vi "Hypervisor_backup.vi"() -> ()   [LabVIEW 2014]
uses:
  Resource Type.ctl
  HypervisorState.ctl
  <vilib>/NI/Tools/String/Tools_String.lvlib
  <userlib>/_OpenG.lib/file/file.llb/Strip Path - Traditional__ogtk.vi
  Sensor Reading.ctl
  Resource.ctl
panel:
  out "Terminal":string
  in  "Module DataType 2":T1
  in  "Cancel Button":bool
  in  "Load Settings":bool
  in  "Module DataType":T1
  in  "Config File":path=path "C:/developer/New Model/config.txt"
  in  "Sensor Reading 3":T3
  in  "Sensor Reading 2":T3
  in  "Hypervisor State":T4=enum."Hypervisor.Sleeping"
  # "This is the hypervisor VI - it reads in a config file and loads the sub-VI's dictated in it asynchronously."
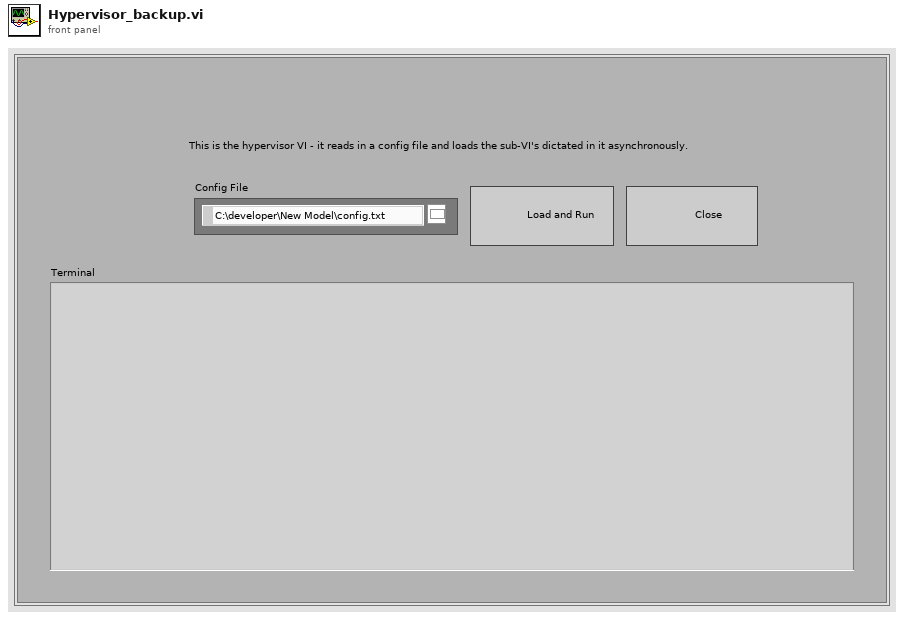
[diagram p1: front panel]
types:
  T1 = typedef "Resource.ctl" = cluster{"Module Name":string, "Message Queue":refnum<queue>, "Resource Type":T2, "Current State":enum16{"Invalid", "InMemory", "Running", "Paused", "Error", ""}, "Data Queue":refnum<queue>, "VI Reference":refnum<vi>}
  T2 = typedef "Resource Type.ctl" = enum16{"Consumer", "Producer", "Observer"}
  T3 = typedef "Sensor Reading.ctl" = cluster{"Sensor Name":string, "Timestamp":string, "Data Chunk":string}
  T4 = typedef "HypervisorState.ctl" = enum16{"Hypervisor.Error", "Hypervisor.Sleeping", "Hypervisor.Loaded", "Hypervisor.Booting", "Hypervisor.Testing", "Hypervisor.Calibrating", "Hypervisor.Running"}
  T5 = enum16{"Invalid", "InMemory", "Running", "Paused", "Error", ""}
  T6 = typedef "Config Data.ctl" = cluster{"Tower ID":string, "Access Password":string}
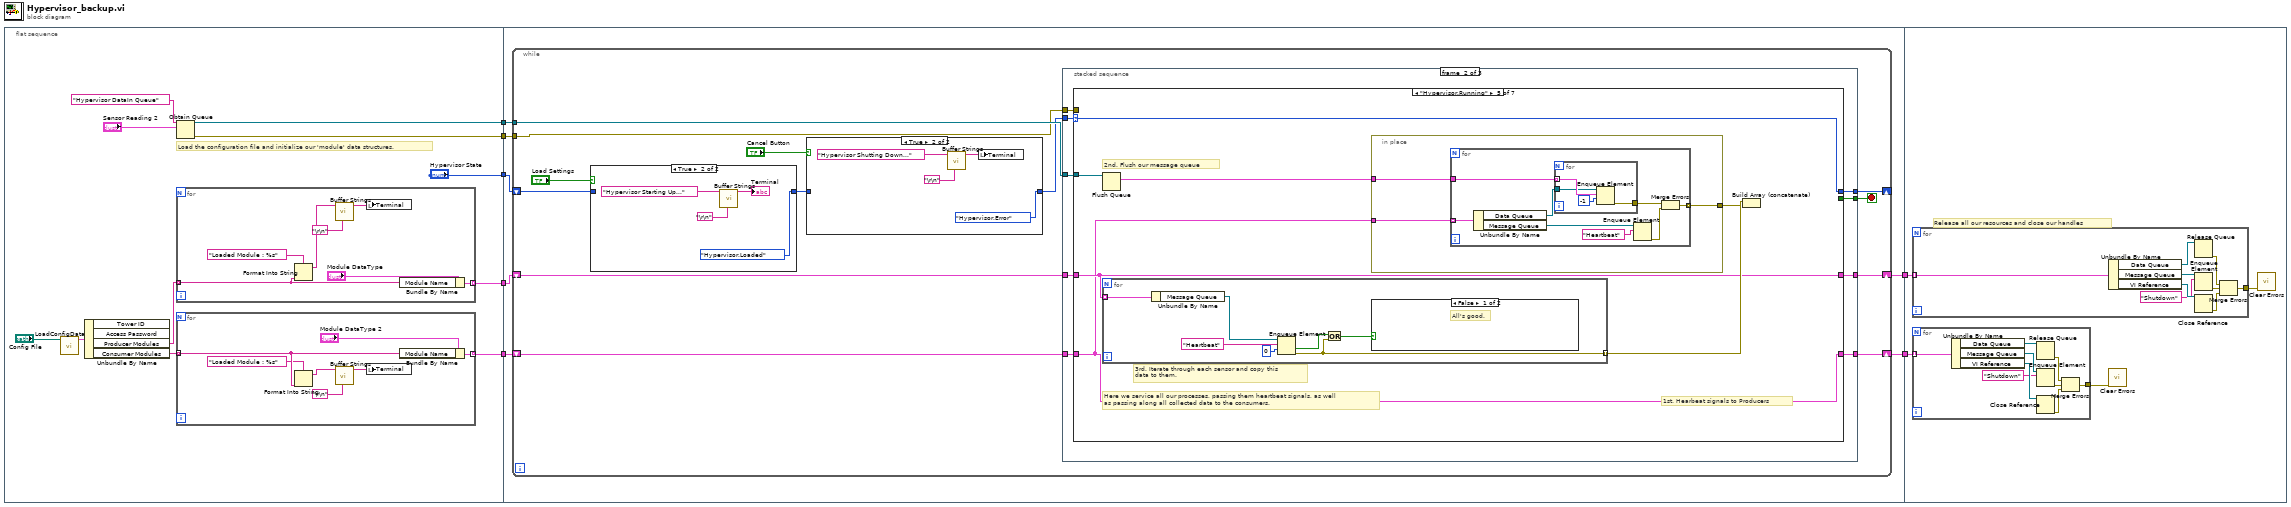
[diagram p0: block diagram]
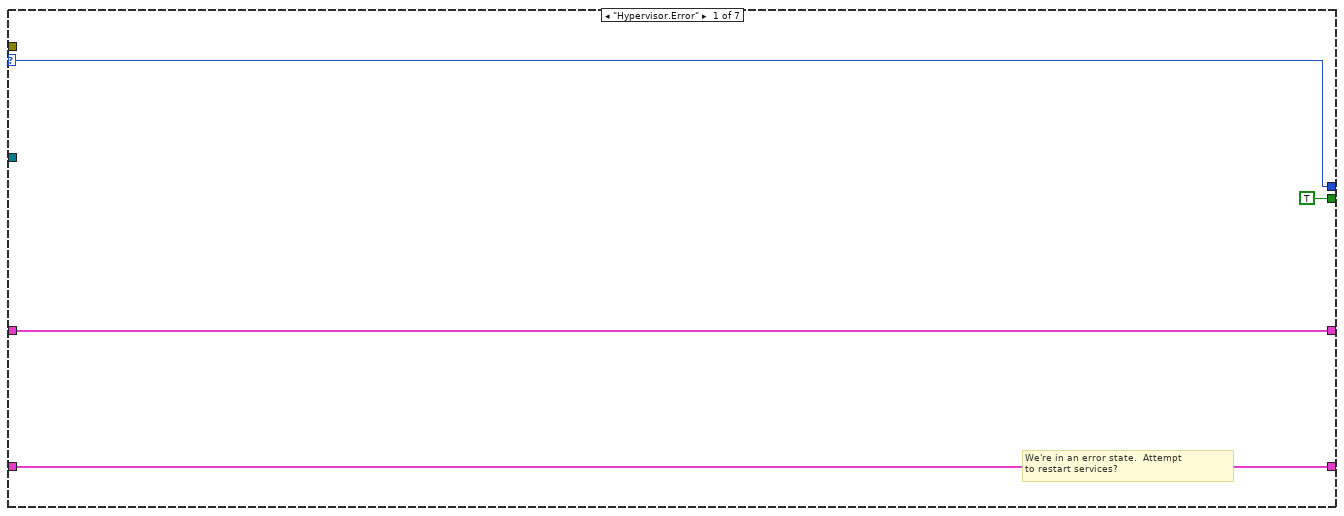
[diagram p5: hidden frame]
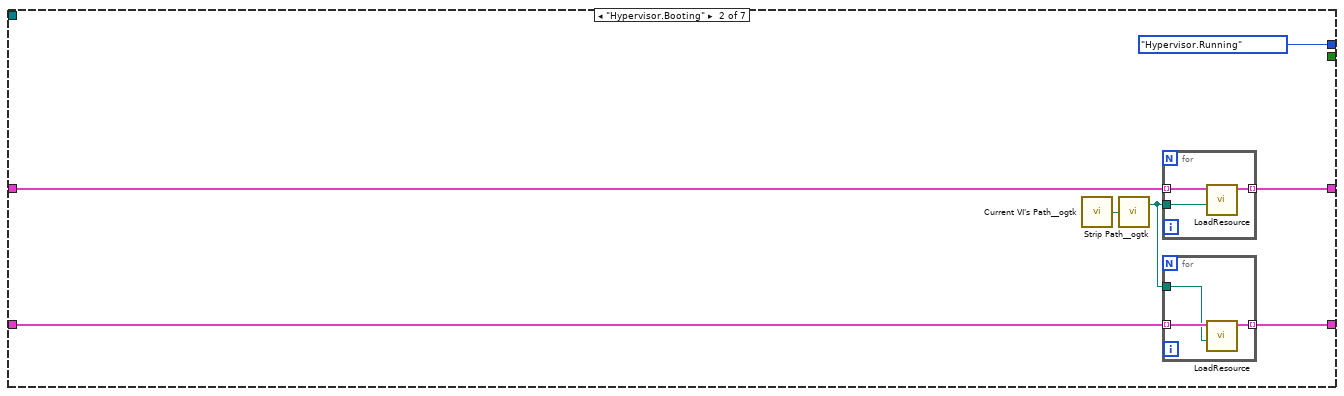
[diagram p6: hidden frame]
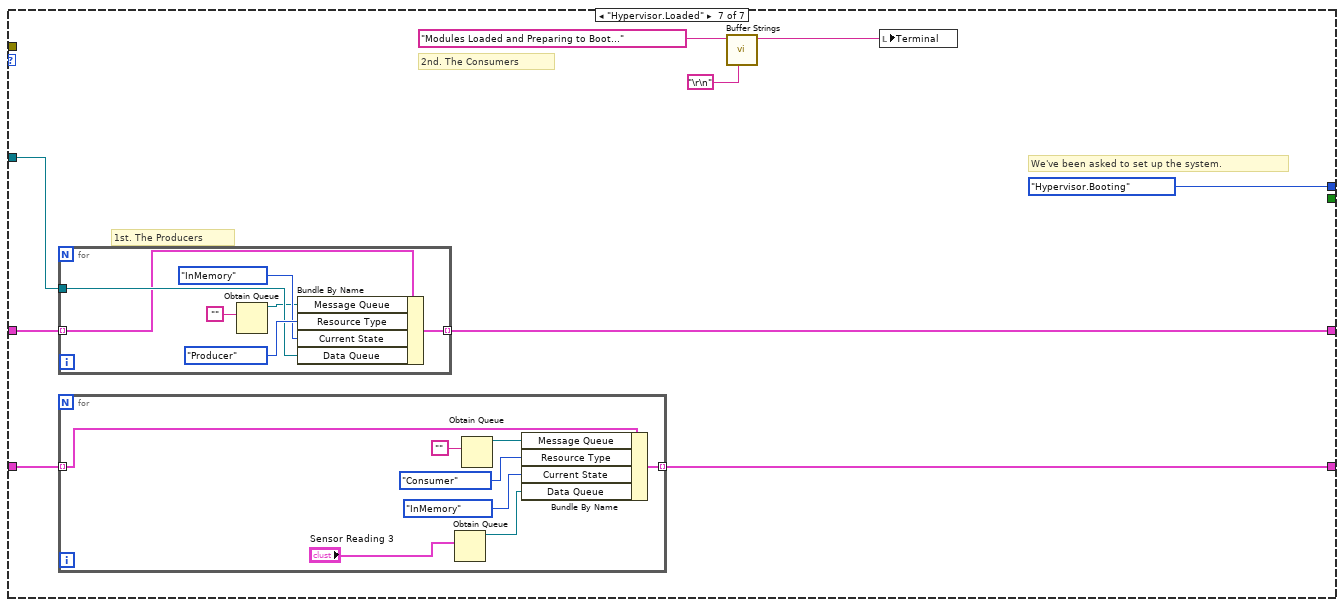
[diagram p11: hidden frame]
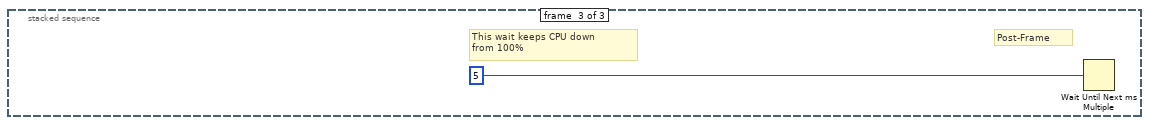
[diagram p12: hidden frame]
diagram:
  n1 = flat-sequence {
    tunnel: ["Hypervisor State"] -> w7
    tunnel: [w10] -> w6
    tunnel: [w8] -> w5
    tunnel: [w16] -> w4
    tunnel: [w15] -> w3
    tunnel: w7 -> [w39]
    tunnel: w6 -> [w38]
    tunnel: w5 -> [w37]
    tunnel: w4 -> [w36]
    tunnel: w3 -> [w35]
    tunnel: [w34] -> w2
    tunnel: [w33] -> w1
    tunnel: w2 -> [w155]
    tunnel: w1 -> [w154]
    frame #0 {
      # "Load the configuration file and initialize our 'module' data structures."
      n2 = call "LoadConfigData.vi"("Config File in"="Config File") -> ("Config Data out"=w12:T6)  [unwired: 10 in]
      n3 = Unbundle By Name(w12) -> ("Producer Modules"=w11:string[], "Consumer Modules"=w9:string[])  [unwired: 2 out]
      n4 = Obtain Queue(name (unnamed)="Hypervisor DataIn Queue", element data type="Sensor Reading 2") -> (queue out=w16:refnum<queue>, error out=w15:errorcluster)  [unwired: 3 in, 1 out]
      n5 = for {
        tunnel: w11 -> [w29] mode=indexing
        tunnel: [w31] -> w10 mode=indexing
        n6 = Format Into String(format string="Loaded Module : %s", w29) -> (resulting string=w28:string)  [unwired: 2 in, 1 out]
        n7 = call <vilib>:"Buffer Strings.vi"("Insert between Strings (\"\")"="\r\n", "new string"=w28) -> ("buffered string series"=w27:string)  [unwired: 9 in]
        n8 = local write "Terminal"(w27) -> ()
        n9 = Bundle By Name(cluster="Module DataType", "Module Name"=w29) -> (w31:T1)
      }
      n10 = for {
        tunnel: w9 -> [w22] mode=indexing
        tunnel: [w24] -> w8 mode=indexing
        n11 = Format Into String(format string="Loaded Module : %s", w22) -> (resulting string=w23:string)  [unwired: 2 in, 1 out]
        n12 = call <vilib>:"Buffer Strings.vi"("Insert between Strings (\"\")"="\r\n", "new string"=w23) -> ("buffered string series"=w20:string)  [unwired: 9 in]
        n13 = local write "Terminal"(w20) -> ()
        n14 = Bundle By Name(cluster="Module DataType 2", "Module Name"=w22) -> (w24:T1)
      }
    }
    frame #1 {
      n15 = while {
        tunnel: w36 -> [w50]
        tunnel: w35 -> [w49]
        shift-right: [w48] -> w34
        shift-left: w38 -> [w52]
        shift-right: [w47] -> w33
        shift-left: w37 -> [w51]
        shift-right: [w46] -> _
        shift-left: w39 -> [w44]
        stop <- w45 stop-if-true
        n16 = case shown="True" "Load Settings" {
          tunnel: w44 -> [w58 _]
          tunnel: [w58 HypervisorState."Hypervisor.Loaded" ("Hypervisor State")] -> w42
          frame False {
          }
          frame True {
            n17 = call <vilib>:"Buffer Strings.vi"("Insert between Strings (\"\")"="\r\n", "new string"="Hypervisor Starting Up...") -> ("buffered string series"=→"Terminal":string)  [unwired: 9 in]
          }
        }
        n18 = case shown="True" "Cancel Button" {
          tunnel: w42 -> [w53 _]
          tunnel: [w53 HypervisorState."Hypervisor.Error" ("Hypervisor State")] -> w41
          frame False {
          }
          frame True {
            n19 = call <vilib>:"Buffer Strings.vi"("Insert between Strings (\"\")"="\r\n", "new string"="Hypervisor Shutting Down...") -> ("buffered string series"=w54:string)  [unwired: 9 in]
            n20 = local write "Terminal"(w54) -> ()
          }
        }
        n21 = stacked-sequence {
          tunnel: w41 -> [_ w64 _]
          tunnel: w52 -> [_ w71 _]
          tunnel: w51 -> [_ w70 _]
          tunnel: w50 -> [_ w69 _]
          tunnel: w49 -> [_ w68 _]
          tunnel: [_ w67 _] -> w48
          tunnel: [_ w66 _] -> w47
          tunnel: [_ w65 _] -> w46
          tunnel: [_ w63 _] -> w45
          frame #0 {
            # "Pre-Frame"
          }
          frame #1 {
            n22 = case shown="\"Hypervisor.Running\"" w64 {
              selector: w64 -> [w73 _ w89 w92 w98 w124 _]
              tunnel: w71 -> [w75 w82 w91 w94 w97 w126 w135]
              tunnel: w70 -> [w74 w79 w90 w93 w96 w125 w132]
              tunnel: w69 -> [_ _ _ _ w101 _ w134]
              tunnel: w68 -> [_ _ _ _ _ _ _]
              tunnel: [w75 w80 w91 w94 w97 w126 w133] -> w67
              tunnel: [w74 w77 w90 w93 w96 w125 w131] -> w66
              tunnel: [w73 HypervisorState."Hypervisor.Running" ("Hypervisor State") w89 w92 w98 w124 HypervisorState."Hypervisor.Booting" ("Hypervisor State")] -> w65
              tunnel: [TRUE _ _ _ _ _ _] -> w63
              frame "Hypervisor.Error" {
                # "We're in an error state.  Attempt\nto restart services?"
              }
              frame "Hypervisor.Booting" {
                n23 = call <userlib>:"Current VI's Path__ogtk.vi"() -> ("Current VI's Path (+ Relative)"=w81:path)  [unwired: 1 in]
                n24 = call-poly <userlib>:"Strip Path__ogtk.vi"("path"=w81) -> ("stripped path"=w78:path)  [unwired: 1 out]
                n25 = for {
                  tunnel: w82 -> [w88] mode=indexing
                  tunnel: w78 -> [w87]
                  tunnel: [w86] -> w80 mode=indexing
                  n26 = call "LoadResource.vi"("Module Root"=w87, "Resource in"=w88) -> ("Resource out"=w86:T1)  [unwired: 8 in, 1 out]
                }
                n27 = for {
                  tunnel: w79 -> [w85] mode=indexing
                  tunnel: w78 -> [w84]
                  tunnel: [w83] -> w77 mode=indexing
                  n28 = call "LoadResource.vi"("Module Root"=w84, "Resource in"=w85) -> ("Resource out"=w83:T1)  [unwired: 8 in, 1 out]
                }
              }
              frame "Hypervisor.Testing" {
              }
              frame "Hypervisor.Calibrating" {
              }
              frame "Hypervisor.Running" {
                # "3rd. Iterate through each sensor and copy this\ndata to them."
                # "2nd. Flush our message queue"
                # "1st. Hearbeat signals to Producers"
                # "Here we service all our processes, passing them heartbeat signals, as well\nas passing along all collected data to the consumers."
                n29 = Flush Queue(queue=w101) -> (remaining elements=w95:T3[])  [unwired: 1 in, 2 out]
                n30 = for {
                  tunnel: w97 -> [w123] mode=indexing
                  tunnel: [w117] -> w100 mode=indexing
                  n31 = Unbundle By Name(w123) -> ("Message Queue"=w122:refnum<queue>)
                  n32 = Enqueue Element(queue=w122, element="Heartbeat", timeout in ms (-1)=0) -> (timed out?=w119:bool, error out=w117:errorcluster)  [unwired: 1 in, 1 out]
                  n33 = Or(x=w119, y=w117) -> (x .or. y?=w118:bool)
                  n34 = case shown="False" w118 {
                    frame False {
                      # "All's good."
                    }
                    frame True {
                      # "Log A Warning"
                    }
                  }
                }
                n35 = in-place {
                  in-place-border: w96 -> [w104]
                  in-place-border: w95 -> [w103]
                  in-place-border: [w102] -> w99
                  n36 = for {
                    tunnel: w104 -> [w111] mode=indexing
                    tunnel: w103 -> [w112]
                    tunnel: [w105] -> w102 mode=indexing
                    n37 = Unbundle By Name(w111) -> ("Data Queue"=w110:refnum<queue>, "Message Queue"=w109:refnum<queue>)
                    n38 = for {
                      tunnel: w112 -> [w116] mode=indexing
                      tunnel: w110 -> [w115]
                      tunnel: [w113] -> w107
                      n39 = Enqueue Element(queue=w115, element=w116, timeout in ms (-1)=-1) -> (error out=w113:errorcluster)  [unwired: 1 in, 2 out]
                    }
                    n40 = Enqueue Element(queue=w109, element="Heartbeat") -> (error out=w106:errorcluster)  [unwired: 2 in, 2 out]
                    n41 = Merge Errors(w107, w106) -> (w105:errorcluster)
                  }
                }
                n42 = Build Array (concatenate)(w100, w99) -> ()  [unwired: 1 out]
              }
              frame "Hypervisor.Sleeping" {
                # "Do Nothing."
              }
              frame "Hypervisor.Loaded" {
                # "2nd. The Consumers"
                # "1st. The Producers"
                # "We've been asked to set up the system."
                n43 = for {
                  tunnel: w135 -> [w145] mode=indexing
                  tunnel: [w148] -> w133 mode=indexing
                  tunnel: w134 -> [w147]
                  n44 = Obtain Queue(element data type="") -> (queue out=w144:refnum<queue>)  [unwired: 4 in, 2 out]
                  n45 = Bundle By Name(cluster=w145, "Message Queue"=w144, "Resource Type"=Resource_Type."Producer", "Current State"=T5."InMemory", "Data Queue"=w147) -> (w148:T1)
                }
                n46 = for {
                  tunnel: [w141] -> w131 mode=indexing
                  tunnel: w132 -> [w138] mode=indexing
                  n47 = Obtain Queue(element data type="Sensor Reading 3") -> (queue out=w137:refnum<queue>)  [unwired: 4 in, 2 out]
                  n48 = Obtain Queue(element data type="") -> (queue out=w139:refnum<queue>)  [unwired: 4 in, 2 out]
                  n49 = Bundle By Name(cluster=w138, "Message Queue"=w139, "Resource Type"=Resource_Type."Consumer", "Current State"=T5."InMemory", "Data Queue"=w137) -> (w141:T1)
                }
                n50 = call <vilib>:"Buffer Strings.vi"("Insert between Strings (\"\")"="\r\n", "new string"="Modules Loaded and Preparing to Boot...") -> ("buffered string series"=w127:string)  [unwired: 9 in]
                n51 = local write "Terminal"(w127) -> ()
              }
            }
          }
          frame #2 {
            # "This wait keeps CPU down\nfrom 100%"
            # "Post-Frame"
            n52 = Wait Until Next ms Multiple(millisecond multiple=u32 5) -> ()  [unwired: 1 out]
          }
        }
      }
    }
    frame #2 {
      # "Release all our resources and close our handles"
      n53 = for {
        tunnel: w155 -> [w173] mode=indexing
        tunnel: [w168] -> w153
        n54 = Unbundle By Name(w173) -> ("Data Queue"=w172:refnum<queue>, "Message Queue"=w167:refnum<queue>, "VI Reference"=w171:refnum<vi>)
        n55 = Release Queue(queue=w172) -> (error out=w170:errorcluster)  [unwired: 2 in, 2 out]
        n56 = Enqueue Element(queue=w167, element="Shutdown") -> (error out=w166:errorcluster)  [unwired: 2 in, 2 out]
        n57 = Close Reference(reference=w171) -> (error out=w169:errorcluster)  [unwired: 1 in]
        n58 = Merge Errors(w170, w166, w169) -> (w168:errorcluster)
      }
      n59 = for {
        tunnel: w154 -> [w164] mode=indexing
        tunnel: [w159] -> w152
        n60 = Unbundle By Name(w164) -> ("Data Queue"=w163:refnum<queue>, "Message Queue"=w158:refnum<queue>, "VI Reference"=w162:refnum<vi>)
        n61 = Release Queue(queue=w163) -> (error out=w161:errorcluster)  [unwired: 2 in, 2 out]
        n62 = Enqueue Element(queue=w158, element="Shutdown") -> (error out=w156:errorcluster)  [unwired: 2 in, 2 out]
        n63 = Close Reference(reference=w162) -> (error out=w160:errorcluster)  [unwired: 1 in]
        n64 = Merge Errors(w161, w156, w160) -> (w159:errorcluster)
      }
      n65 = call <vilib>:"Clear Errors.vi"("error in (no error)"=w152) -> ()  [unwired: 5 in, 2 out]
      n66 = call <vilib>:"Clear Errors.vi"("error in (no error)"=w153) -> ()  [unwired: 5 in, 2 out]
    }
  }
